vi "PH_PowerUnit_BaseClass.ProcEvents.vi"(0 "i ref in":refnum<vi>, 5 "error in (no error)":errorcluster) -> (14 "i ref out":refnum<vi>, 19 "error out":errorcluster)   [LabVIEW 2014, in "PH_PowerUnit_BaseClass.lvlib"]
doc: "This method is used to define the events the object will listen to. Add your own events here."
uses:
  PH_PowerUnit_BaseClass.lvlib
  CS_Core/BaseProcess/BaseProcess.event definition.ctl
  CS_Core/CAEObj/CAEObj.event definition.ctl
  CS_Core/BaseProcess/BaseProcess.descriptor string definition.ctl
  CS_Core/BaseProcess/BaseProcess.lvlib
  CS_Core/CAEObj/CAEObj.lvlib
  PH_Common/PH_Common.lvlib
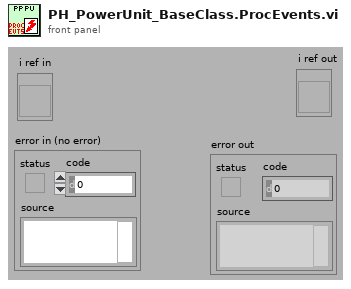
[diagram p1: front panel]
types:
  T1 = typedef "BaseProcess.lvlib/BaseProcess.event definition.ctl" = cluster{"CAEEvtDef":T2, "Data Descriptor":T3}
  T2 = typedef "CAEObj.lvlib/CAEObj.event definition.ctl" = cluster{"URL":string, "enable":bool, "ignoreResID":bool}
  T3 = typedef "BaseProcess.lvlib/BaseProcess.descriptor string definition.ctl" = string
  T4 = typedef "PH_PowerUnit_BaseClass.lvlib/PH_PowerUnit_BaseClass.i attribute.ctl" = cluster{"Constructor finished":bool, "PU":cluster{"In use":bool, "Service ID in use":i32, "GUI Ref":refnum<vi>}, "Enabling":cluster{"State":T5, "GUI Ref":refnum<vi>}, "Timing":cluster{"Last Shot":dbl, "Time between Shots [Sec]":dbl, "Waiting Time over?":bool, "Service ID Waiting Time":i32, "GUI Ref":refnum<vi>, "Instance":cluster{"Status":T6, "linked?":bool, "GUI Ref":refnum<vi>}}, "Sequencer":cluster{"SM State":string, "GUI Ref":refnum<vi>, "linked":bool}, "Subscribed Trendmssgs":cluster{"Tagname":string, "Status":T6, "linked?":bool, "Shot Condition":T6, "GUI Ref":refnum<vi>}[], "PP PU":T7, "Default Voltage (V)":dbl, "GUI Refs":T8, "PSDB data":cluster{"Shot Voltage [V]":dbl, "State TO SM":T9, "Write 2 early":bool}, "State TO SM":T9}
  T5 = typedef "PH_SystemInformation.lvlib/PH_SystemInformationEnabling State.ctl" = i32
  T6 = typedef "PH_StatusHandler.lvlib/PH_StatusHandler.Status.ctl" = i16
  T7 = typedef "PH_PP_Common.lvlib/PH_PP_Common.PUs.ctl" = enum16{"no Info", "PA-19mm-1", "PA-19mm-2", "PA-45mm-PILC", "PA-45mm-MAIN", "MA-PU-1", "MA-PU-2", "MA-PU-3", "MA-PU-4", "MA-PU-5", "MA-PU-6", "MA-FR", "MA-PILC", "PA-45mm-DP"}
  T8 = typedef "PH_PowerUnit_BaseClass.lvlib/PH_PowerUnit_BaseClass.GUI Refs.ctl" = cluster{"Delete Inst":refnum<vi>, "State TO SM":refnum<vi>, "State SM":refnum<vi>, "Fire":refnum<vi>}
  T9 = typedef "PH_PowerUnit_BaseClass.lvlib/PH_PowerUnit_BaseClass.SM States.ctl" = enum16{".", "Stand by", "Switch PU on", "Configure", "Set Default Voltage", "Set STANDBY", "Set READY", "Wait for Shot Cmd", "Open Dump Rods", "Open Ross Relais", "Close Ross Relais", "Switch PSU on", "Switch PSU off", "Charge", "Switch GD Channel on", "Close Dump Rods", "Rods-TO", "RR-TO", "PSU-TO", "Trigger-TO"}
  T10 = cluster{"Tagname":string, "Status":T6, "linked?":bool, "Shot Condition":T6, "GUI Ref":refnum<vi>}[]
  T11 = typedef "PH_Common.lvlib/PH_DIM.Event Declarer.ctl" = cluster{"Service Name":string, "Selector":string}
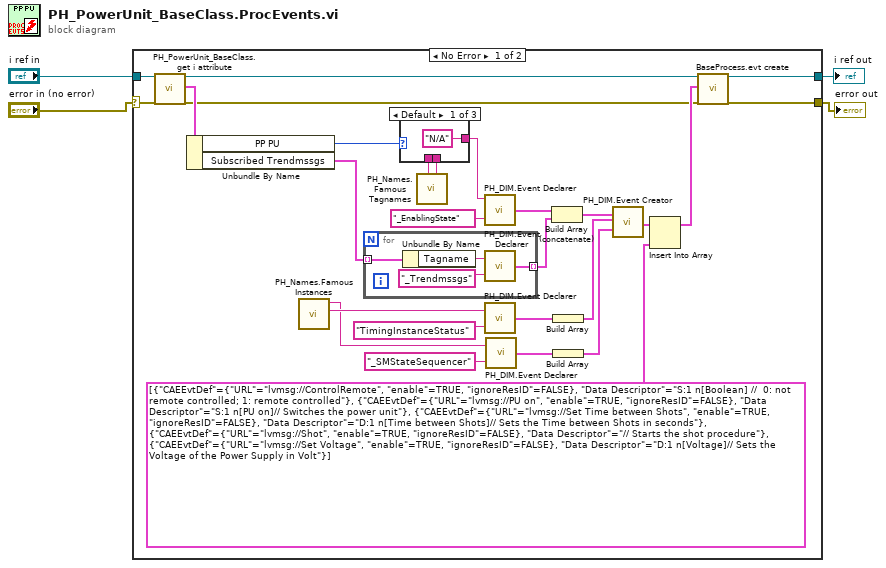
[diagram p0: block diagram]
diagram:
  n1 = case shown="No Error" "error in (no error)" {
    selector: "error in (no error)" -> [w25 w39]
    tunnel: "i ref in" -> [w31 w40]
    tunnel: [w30 w40] -> w3
    tunnel: [w29 w39] -> w2
    frame No Error {
      n2 = call "PH_PowerUnit_BaseClass.get i attribute.vi"("i ref in"=w31, "error in (no error)"=w25) -> ("i ref out"=w16:refnum<vi>, "i attribute"=w28:T4, "error out"=w15:errorcluster)  [unwired: 15 in]
      n3 = Unbundle By Name(w28) -> ("PP PU"=w8:T7, "Subscribed Trendmssgs"=w14:T10)
      n4 = call "PH_Names.Famous Instances.vi"() -> ("Sequencer"=w5:string, "Timing"=w6:string)  [unwired: 7 in, 2 out]
      n5 = for {
        tunnel: [w37] -> w13 mode=indexing
        tunnel: w14 -> [w36] mode=indexing
        n6 = Unbundle By Name(w36) -> ("Tagname"=w35:string)
        n7 = call "PH_DIM.Event Declarer.vi"("Selector"="_Trendmssgs", "Service Name"=w35) -> ("declared DIM Event"=w37:T11)
      }
      n8 = call "PH_Names.Famous Tagnames.vi"() -> ("PreAmp Enabling.DIM Service Name"=w7:string, "MainAmp Enabling.DIM Service Name"=w10:string)  [unwired: 2 in, 7 out]
      n9 = case shown="Default" w8 {
        tunnel: ["N/A" ("MainAmp Enabling.DIM Service Name") w33 w34] -> w9
        tunnel: w7 -> [_ w33 _]
        tunnel: w10 -> [_ _ w34]
        frame Default {
        }
        frame "PA-19mm-1".."PA-45mm-MAIN", "PA-45mm-DP" {
        }
        frame "MA-PU-1".."MA-PILC" {
        }
      }
      n10 = call "PH_DIM.Event Declarer.vi"("Selector"="_EnablingState", "Service Name"=w9) -> ("declared DIM Event"=w23:T11)
      n11 = call "PH_DIM.Event Declarer.vi"("Selector"="TimingInstanceStatus", "Service Name"=w6) -> ("declared DIM Event"=w17:T11)
      n12 = call "PH_DIM.Event Declarer.vi"("Selector"="_SMStateSequencer", "Service Name"=w5) -> ("declared DIM Event"=w21:T11)
      n13 = Build Array (concatenate)(w23, w13) -> (w22:T11[])
      n14 = Build Array(w17) -> (w11:T11[])
      n15 = Build Array(w21) -> (w19:T11[])
      n16 = call "PH_DIM.Event Creator.vi"("Trendmessage Services"=w22, "Status Services"=w11, "SM State Services"=w19) -> ("DIM Service Events"=w27:T1[])  [unwired: 16 in]
      n17 = Insert Into Array(array=w27, new element=T1[] [{"CAEEvtDef"={"URL"="lvmsg://ControlRemote", "enable"=TRUE, "ignoreResID"=FALSE}, "Data Descriptor"="S:1 n[Boolean] //  0: not remote controlled; 1: remote controlled"}, {"CAEEvtDef"={"URL"="lvmsg://PU on", "enable"=TRUE, "ignoreResID"=FALSE}, "Data Descriptor"="S:1 n[PU on]// Switches the power unit"}, {"CAEEvtDef"={"URL"="lvmsg://Set Time between Shots", "enable"=TRUE, "ignoreResID"=FALSE}, "Data Descriptor"="D:1 n[Time between Shots]// Sets the Time between Shots in seconds"}, {"CAEEvtDef"={"URL"="lvmsg://Shot", "enable"=TRUE, "ignoreResID"=FALSE}, "Data Descriptor"="// Starts the shot procedure"}, {"CAEEvtDef"={"URL"="lvmsg://Set Voltage", "enable"=TRUE, "ignoreResID"=FALSE}, "Data Descriptor"="D:1 n[Voltage]// Sets the Voltage of the Power Supply in Volt"}] ("new events")) -> (w24:T1[])  [unwired: 1 in]
      n18 = call "BaseProcess.evt create.vi"("i ref in"=w16, "newEvents"=w24, "error in (no error)"=w15) -> ("i ref out"=w30:refnum<vi>, "error out"=w29:errorcluster)  [unwired: 13 in, 2 out]
    }
    frame Error {
    }
  }
  "i ref out" <- w3
  "error out" <- w2
